vi "ScpChTrSetEnabled.vi"(8 "error in (no error)":errorcluster, 9 "TrigEnable":bool, 10 "wCh":u16, 11 "hDevice":u32) -> (0 "error out":errorcluster, 1 "TrEnbaled?":bool, 2 "wCh out":u16, 3 "hDevice out":u32)   [LabVIEW 2018, in "LibTiePie.lvlib"]
uses:
  LibTiePie.lvlib
  LabViewHS4/libtiepie.dll
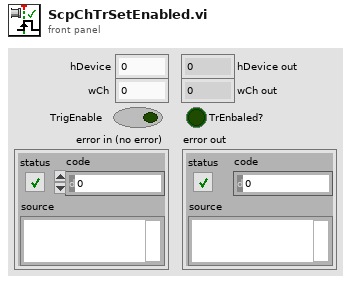
[diagram p1: front panel]
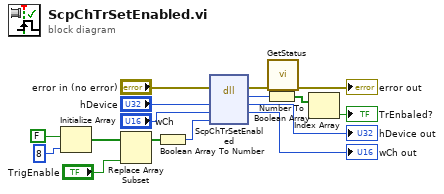
[diagram p0: block diagram]
diagram:
  n1 = Initialize Array(FALSE, 8 ("dimension size")) -> (w11:bool[])
  n2 = Replace Array Subset(array=w11, new element="TrigEnable") -> (w9:bool[])  [unwired: 1 in]
  n3 = Boolean Array To Number(Boolean array=w9) -> (number=w8:u8)
  n4 = dll-call lib="C:/Users/cwaha/Documents/LabViewHS4/libtiepie.dll" fn="ScpChTrSetEnabled"(error in="error in (no error)", "hDevice"="hDevice", "wCh"="wCh", "bEnabled"=w8) -> (error out=w7:errorcluster, "bTrigEnabled"=w5:u8, "hDevice"=→"hDevice out":u32, "wCh"=→"wCh out":u16)  [unwired: 3 in, 1 out]
  n5 = Number To Boolean Array(number=w5) -> (Boolean array=w4:bool[])
  n6 = call "GetStatus.vi"("error in (no error)"=w7) -> ("error out"=→"error out":errorcluster)  [unwired: 10 in]
  n7 = Index Array(array=w4) -> (element=→"TrEnbaled?":bool)  [unwired: 1 in]
